vi "Generate Cached Images.vi"(8 "error in (no error)":errorcluster, 9 "Button Style":T1=enum."Classic", 10 "Button Size":i32, 11 "object in":refnum<class "Button.lvclass">) -> (0 "error out":errorcluster, 3 "object out":refnum<class "Button.lvclass">)   [LabVIEW 2012, in "Button.lvclass"]
doc: "Generates fresh versions of button images to store in the cache."
uses:
  Button.lvclass
  Type Defs/Button Style.ctl
  Button.lvclass/Button.ctl
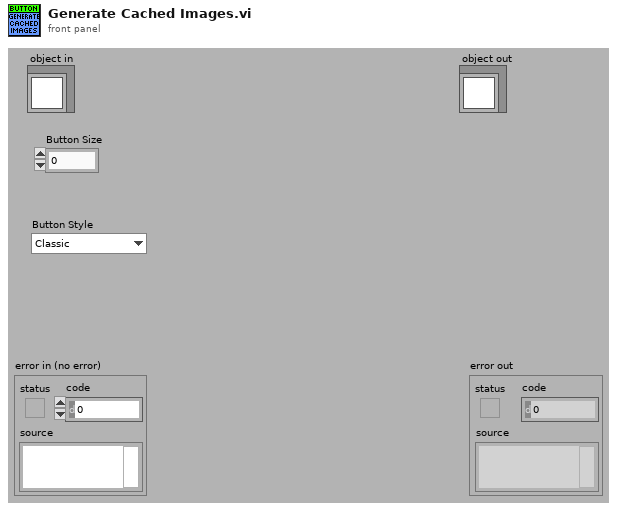
[diagram p1: front panel]
types:
  T1 = typedef "Button.lvclass/Button Style.ctl" = enum16{"System", "Modern", "Classic", "Rounded", "Silver", "Ni Theme", "Metallic"}
  T2 = typedef "imagedata.ctl" = cluster{"image type":i32, "image depth":i32, "image":u8[], "mask":u8[], "colors":u32[], "Rectangle":cluster{"left":i16, "top":i16, "right":i16, "bottom":i16}}
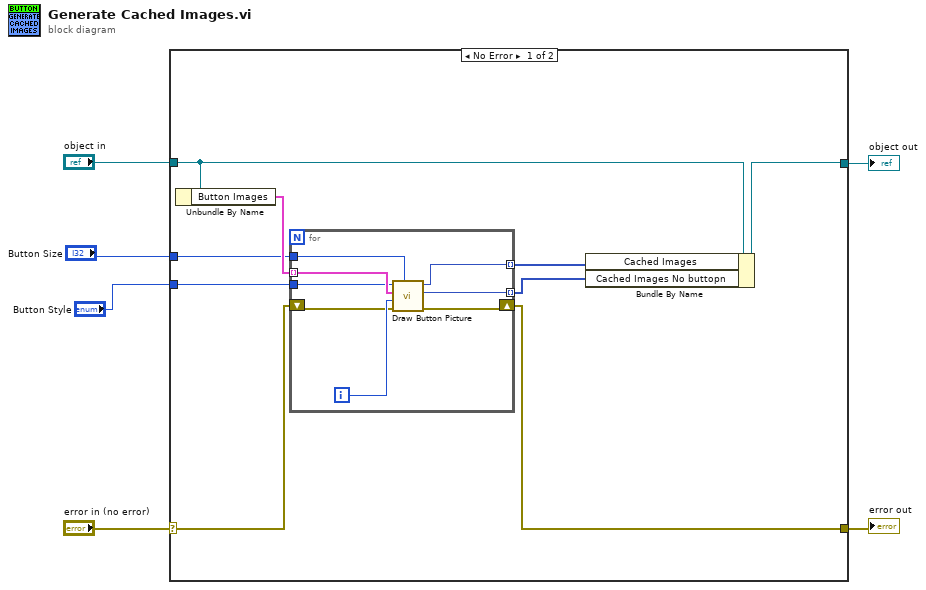
[diagram p0: block diagram]
diagram:
  n1 = case shown="No Error" "error in (no error)" {
    selector: "error in (no error)" -> [w8 w25]
    tunnel: [w7 w25] -> w5
    tunnel: [w15 w24] -> w3
    tunnel: "object in" -> [w14 w24]
    tunnel: "Button Size" -> [w12 _]
    tunnel: "Button Style" -> [w11 _]
    frame No Error {
      n2 = Unbundle By Name(w14) -> ("Button Images"=w13:T2[])
      n3 = for {
        tunnel: w13 -> [w23] mode=indexing
        shift-right: [w21] -> w7
        shift-left: w8 -> [w20]
        tunnel: w12 -> [w19]
        tunnel: w11 -> [w18]
        tunnel: [w17] -> w9 mode=indexing
        tunnel: [w16] -> w10 mode=indexing
        i -> [w22]
        n4 = call "Draw Button Picture.vi"("Button Size"=w19, "error in (no error)"=w20, "Button State"=w22, "image data"=w23, "Button Style"=w18) -> ("error out"=w21:errorcluster, "Image (no button)"=w16:picture, "Picture Out"=w17:picture)  [unwired: 4 in]
      }
      n5 = Bundle By Name(cluster=w14, "Cached Images"=w9, "Cached Images No buttopn"=w10) -> (w15:refnum<class "Button.lvclass">)
    }
    frame Error {
    }
  }
  "error out" <- w5
  "object out" <- w3
